vi "Collision test simple.vi"(3 "Octree for query triangles":T2[](array[typedef]), 4 "Query triangles":T1[](array[typedef]), 5 "Triangle to test":T1) -> (0 "Indices of possible triangles":i32[](array[numeric]), 1 "Collision point(s)":sgl[][](array[numeric]), 2 "Collision(s)?":bool)   [LabVIEW 2014]
doc: "This VI returns the first collision found between the test triangle and the query triangles. It does not return the minimum separation vector and distance in the case of no collision."
uses:
  Typedefs/Triangle.ctl
  Typedefs/TreeNodeBox.ctl
  Typedefs/Quad.ctl
  Typedefs/Quadplane enum.ctl
  Subroutines/Edge-Tri intersection test.vi
  Subroutines/Point-in-Tri test.vi
  Subroutines/Edge-Plane intersection test.vi
  Subroutines/Dot product.vi
panel:
  # "PN 03/02/2015, 13/03/2015"
  # "Vertices"
  # "Edges"
  # "Unit normal"
  # "Edge unit normals"
  # "Vertices"
  # "Edges"
  # "Unit normal"
  # "Plane ident."
  # "Vertices"
  # "Edges"
  # "Unit normal"
  # "Plane ident."
  # "Vertices"
  # "Edges"
  # "Unit normal"
  # "Plane ident."
  # "Vertices"
  # "Edges"
  # "Unit normal"
  # "Plane ident."
  # "Vertices"
  # "Edges"
  # "Unit normal"
  # "Plane ident."
  # "Vertices"
  # "Edges"
  # "Unit normal"
  # "Plane ident."
  # "Vertices"
  # "Edges"
  # "Unit normal"
  # "Edge unit normals"
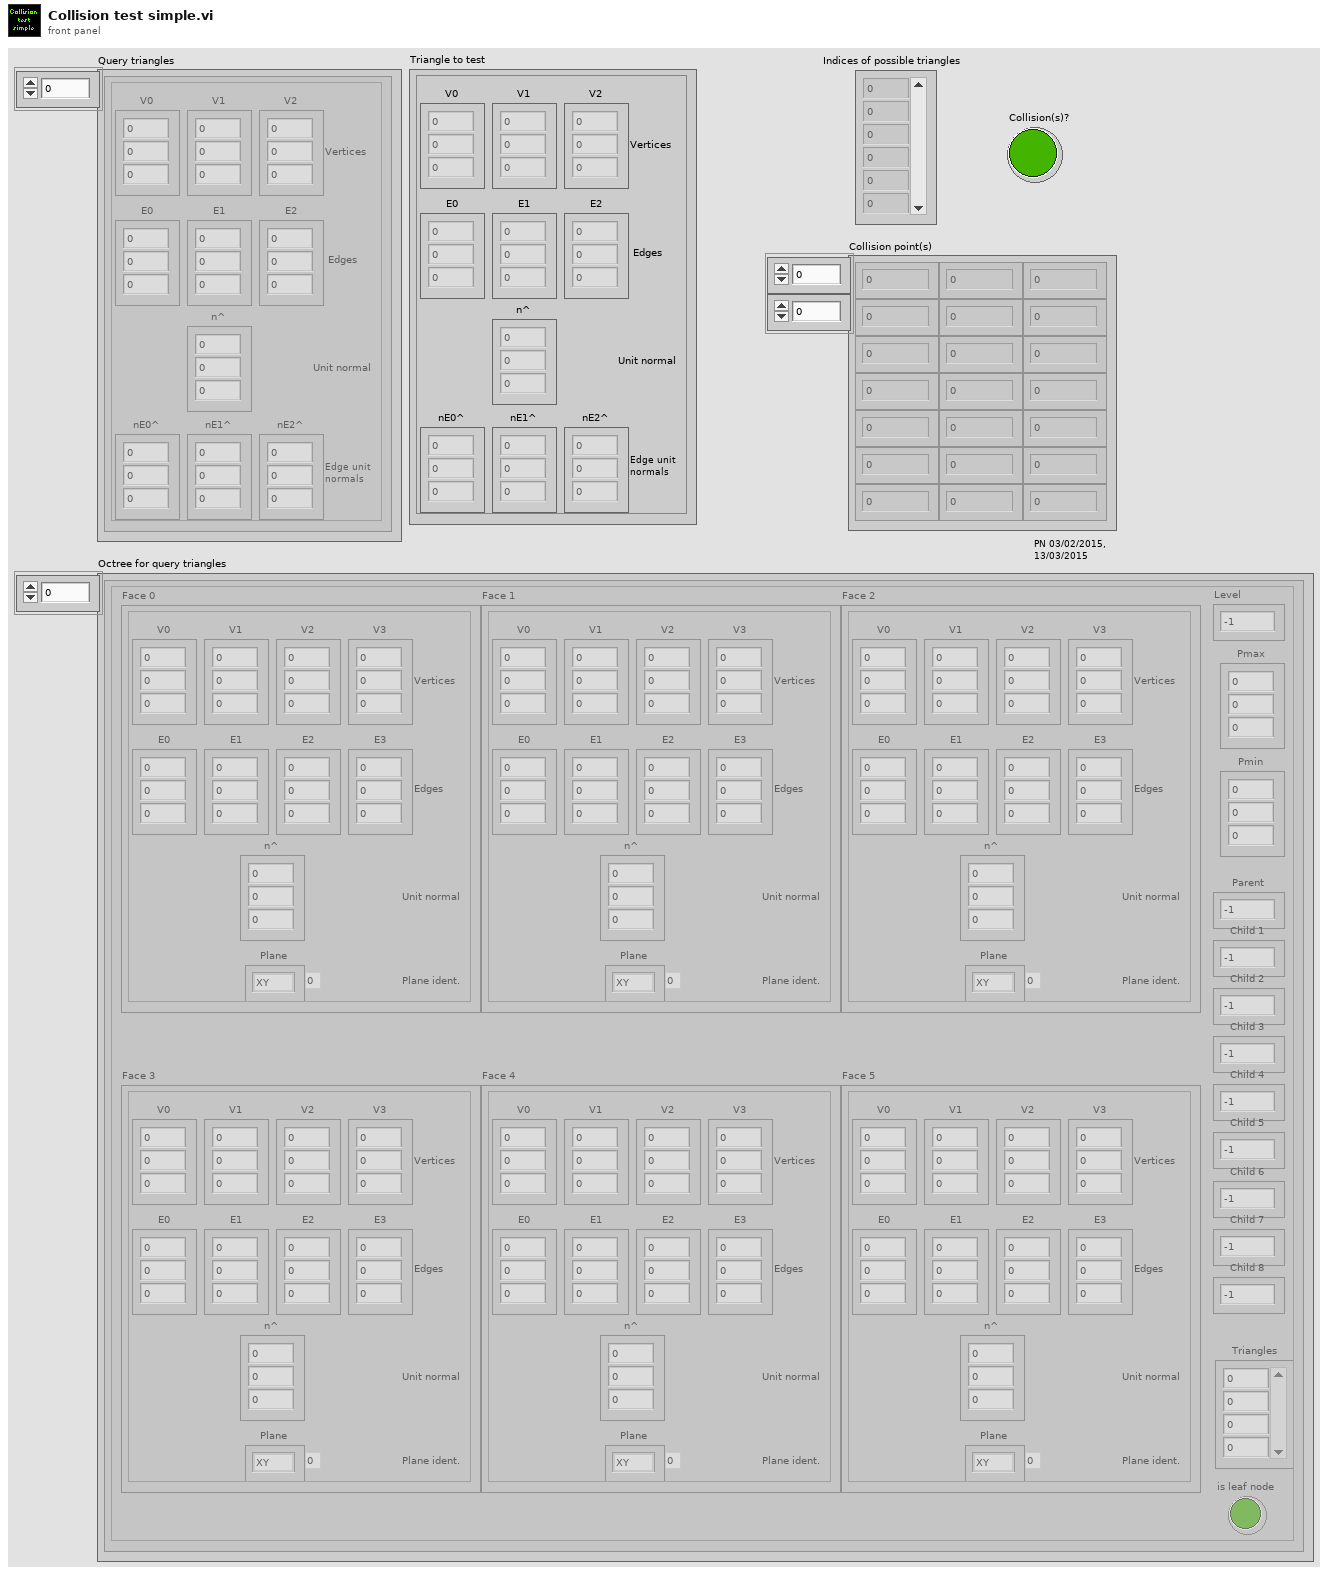
[diagram p1: front panel]
types:
  T1 = typedef "Triangle.ctl" = cluster{"V0":sgl[], "V1":sgl[], "V2":sgl[], "E0":sgl[], "E1":sgl[], "E2":sgl[], "n^":sgl[], "nE0^":sgl[], "nE1^":sgl[], "nE2^":sgl[]}
  T2 = typedef "TreeNodeBox.ctl" = cluster{"Face 0":T3, "Face 1":T3, "Face 2":T3, "Face 3":T3, "Face 4":T3, "Face 5":T3, "Level":i32, "Pmax":sgl[], "Pmin":sgl[], "Parent":i32, "Child 1":i32, "Child 2":i32, "Child 3":i32, "Child 4":i32, "Child 5":i32, "Child 6":i32, "Child 7":i32, "Child 8":i32, "Triangles":i32[], "is leaf node":bool}
  T3 = typedef "Quad.ctl" = cluster{"V0":sgl[], "V1":sgl[], "V2":sgl[], "V3":sgl[], "E0":sgl[], "E1":sgl[], "E2":sgl[], "E3":sgl[], "n^":sgl[], "Plane":T4}
  T4 = typedef "Quadplane enum.ctl" = enum8{"XY", "XZ", "YZ", "-XY", "-XZ", "-YZ"}
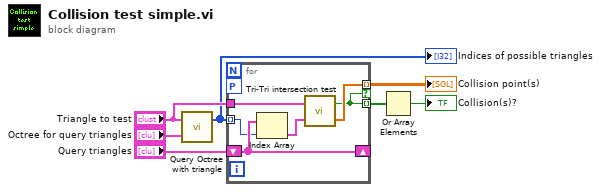
[diagram p0: block diagram]
diagram:
  n1 = call "Query Octree with triangle.vi"("Octree node array"="Octree for query triangles", "Triangle"="Triangle to test") -> ("Indices of possible triangles"=w5:i32[])  [unwired: 1 out]
  "Indices of possible triangles" <- w5
  n2 = for {
    tunnel: "Triangle to test" -> [w9]
    tunnel: w5 -> [w12] mode=indexing
    shift-right: [w13] -> _
    shift-left: "Query triangles" -> [w13]
    tunnel: [w8] -> w3 mode=indexing
    tunnel: [w11] -> w1 mode=indexing if=w8
    workers-P: _ -> [_]
    n3 = Index Array(array=w13, index=w12) -> (element=w10:T1)
    n4 = call "Tri-Tri intersection test.vi"("Triangle 2"=w10, "Triangle 1"=w9) -> ("Intersection point"=w11:sgl[], "Intersection"=w8:bool)
  }
  "Collision point(s)" <- w1
  n5 = Or Array Elements(Boolean array=w3) -> (logical OR=→"Collision(s)?":bool)
